vi "Close.vi"(8 "error in (no error)":errorcluster, 11 "Abstract Sensor in":refnum<class "Abstract Sensor.lvclass">) -> (0 "error out":errorcluster, 3 "Abstract Sensor out":refnum<class "Abstract Sensor.lvclass">)   [LabVIEW 2014, in "Abstract Sensor.lvlib" / "Abstract Sensor.lvclass"]
uses:
  Abstract Sensor.lvclass
  Generic Instrument/Generic Instrument.lvclass
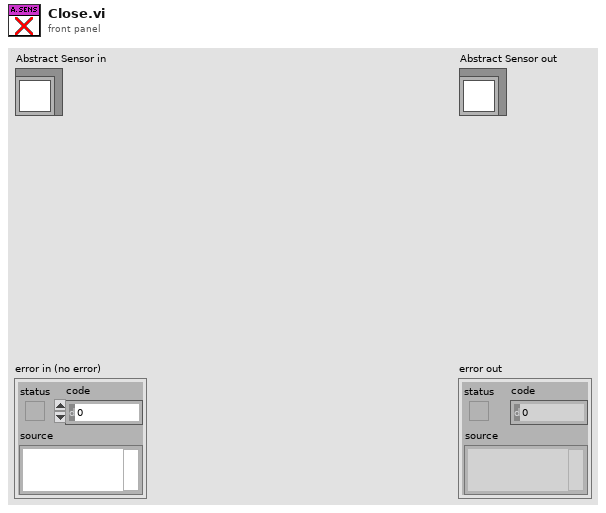
[diagram p1: front panel]
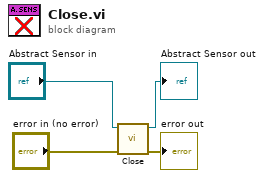
[diagram p0: block diagram]
diagram:
  n1 = call-parent "Close.vi"("error in (no error)"="error in (no error)", "Generic Instrument in"="Abstract Sensor in") -> ("error out"=→"error out":errorcluster, "Generic Instrument out"=→"Abstract Sensor out":refnum<class "Abstract Sensor.lvclass">)  [unwired: 8 in]
